vi "Generate Mouse Click.vi"(8 "error in (no error)":errorcluster) -> (0 "error out":errorcluster)   [LabVIEW 2021, in "Create Measurement Plug-In Client.lvlib"]
uses:
  Create Measurement Plug-In Client.lvlib
  user32.dll
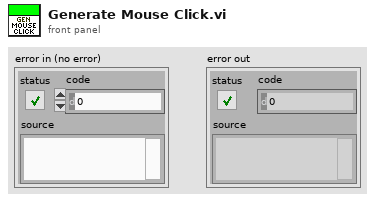
[diagram p1: front panel]
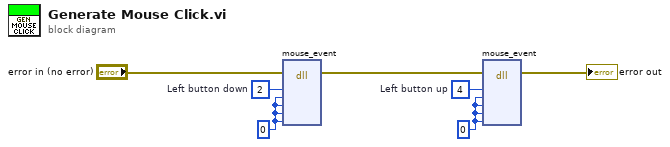
[diagram p0: block diagram]
diagram:
  w4 = u32 0 ("dx")
  w5 = 4  # Left button up
  w2 = u32 0 ("dx")
  w1 = 2  # Left button down
  n1 = dll-call lib="user32.dll" fn="mouse_event" label="Click"(error in="error in (no error)", "dwFlags"=w1, "dx"=w2, "dy"=w2, "dwData"=w2, "dwExtraInfo"=w2) -> (error out=w7:errorcluster)  [unwired: 8 in, 1 out]
  n2 = dll-call lib="user32.dll" fn="mouse_event" label="Release"(error in=w7, "dwFlags"=w5, "dx"=w4, "dy"=w4, "dwData"=w4, "dwExtraInfo"=w4) -> (error out=→"error out":errorcluster)  [unwired: 8 in, 1 out]
